vi "测试应用程序3.vi"() -> ()   [LabVIEW 2022 SP3]
doc: "本VI是为《我和LabVIEW》一书编写的示例。\n关于本书的介绍请参考网页：\nhttp://ruanqizhen.spaces.live.com/blog/cns!5852D4F797C53FB6!4310.entry"
panel:
  out "数据":dbl
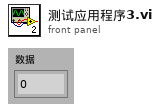
[diagram p1: front panel]
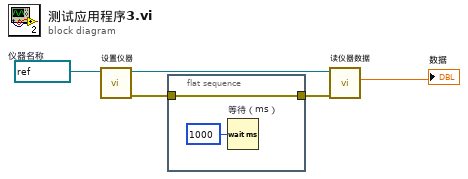
[diagram p0: block diagram]
diagram:
  w3 = refnum<visa-resource-name> "XX仪"  # 仪器名称
  n1 = call "设置仪器.vi"("VISA资源名称"=w3) -> ("error out"=w2:errorcluster, "仪器句柄"=w5:refnum<visa-resource-name>)  [unwired: 1 in, 8 out]
  n2 = flat-sequence {
    tunnel: w2 -> [w6]
    tunnel: [w6] -> w1
    frame #0 {
      n3 = Wait (ms) "等待（ms）"(milliseconds to wait=u32 1000 ("等待时间（毫秒）")) -> ()  [unwired: 1 out]
    }
  }
  n4 = call "读仪器数据.vi"("error in (no error)"=w1, "仪器句柄"=w5) -> ("数据"=→"数据":dbl)  [unwired: 9 out]
